vi "站点编码更新（年月日）.vi"(10 "当前编码信息":string, 11 "站别":string) -> ()   [LabVIEW 2018]
uses:
  <vilib>/Utility/file.llb/Read From Spreadsheet File (string).vi
panel:
  out "错误输出":errorcluster
  out "error out":errorcluster caption="错误输出"
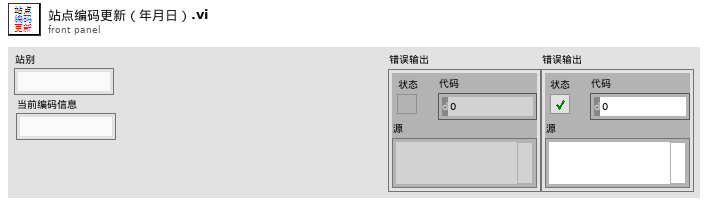
[diagram p1: front panel]
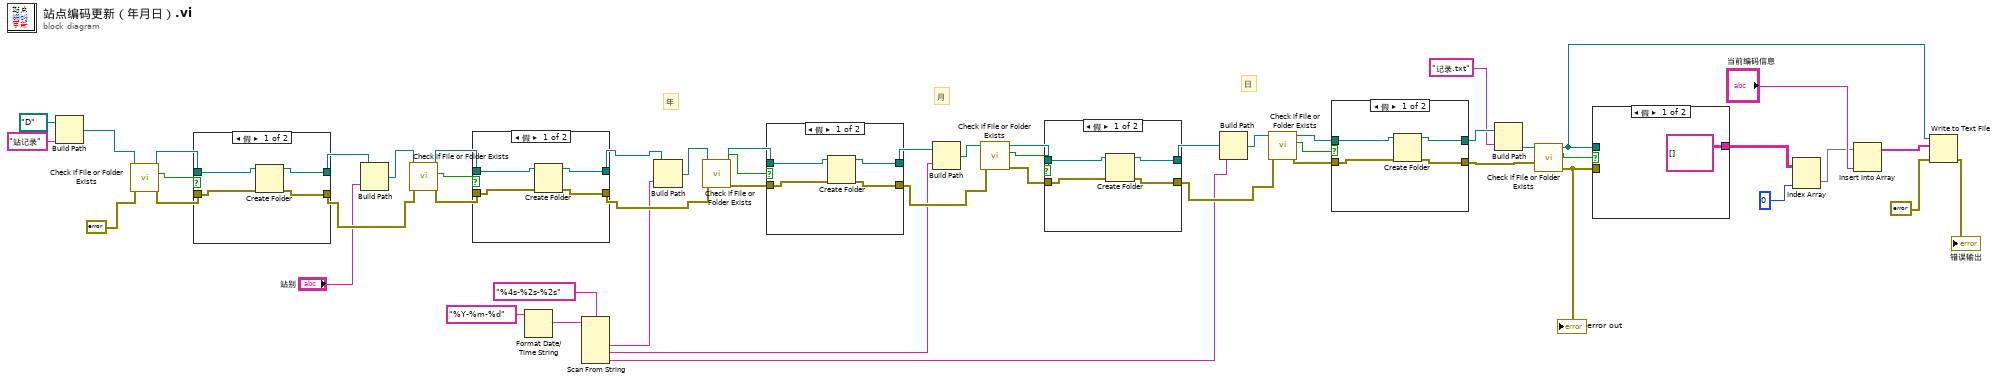
[diagram p0: block diagram]
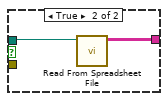
[diagram p2: hidden frame]
diagram:
  # "日"
  # "月"
  # "年"
  n1 = Build Path(base path=path "D:/" ("基路径"), name or relative path="站记录" ("名称或相对路径")) -> (appended path=w50:path)
  n2 = call <vilib>:"Check if File or Folder Exists.vi"("error in (no error)"=errorcluster {"status"=FALSE, "code"=0, "source"=""}, "path"=w50) -> ("error out"=w47:errorcluster, "file or folder exists?"=w49:bool, "dup path"=w48:path)  [unwired: 7 in]
  n3 = case shown="假" w49 {
    tunnel: w48 -> [w56 w58]
    tunnel: w47 -> [w55 w57]
    tunnel: [w54 w58] -> w42
    tunnel: [w53 w57] -> w40
    frame False {
      n4 = Create Folder(path (use dialog)=w56, error in=w55) -> (created path=w54:path, error out=w53:errorcluster)  [unwired: 1 in, 1 out]
    }
    frame True {
    }
  }
  n5 = Build Path(base path=w42, name or relative path="站别") -> (appended path=w41:path)
  n6 = call <vilib>:"Check if File or Folder Exists.vi"("error in (no error)"=w40, "path"=w41) -> ("error out"=w44:errorcluster, "file or folder exists?"=w46:bool, "dup path"=w45:path)  [unwired: 7 in]
  n7 = case shown="假" w46 {
    tunnel: w45 -> [w62 w64]
    tunnel: w44 -> [w61 w63]
    tunnel: [w60 w64] -> w34
    tunnel: [w59 w63] -> w33
    frame False {
      n8 = Create Folder(path (use dialog)=w62, error in=w61) -> (created path=w60:path, error out=w59:errorcluster)  [unwired: 1 in, 1 out]
    }
    frame True {
    }
  }
  n9 = Format Date/Time String(time format string (%c)="%Y-%m-%d" ("时间格式字符串(%c)")) -> (date/time string=w31:string)  [unwired: 2 in]
  n10 = Scan From String(format string="%4s-%2s-%2s" ("格式字符串"), input string=w31) -> (output 1=w29:string, output 2=w22:string, output 3=w15:string)  [unwired: 5 in, 3 out]
  n11 = Build Path(base path=w34, name or relative path=w29) -> (appended path=w35:path)
  n12 = call <vilib>:"Check if File or Folder Exists.vi"("error in (no error)"=w33, "path"=w35) -> ("error out"=w36:errorcluster, "file or folder exists?"=w38:bool, "dup path"=w37:path)  [unwired: 7 in]
  n13 = case shown="假" w38 {
    tunnel: w37 -> [w68 w70]
    tunnel: w36 -> [w67 w69]
    tunnel: [w66 w70] -> w24
    tunnel: [w65 w69] -> w23
    frame False {
      n14 = Create Folder(path (use dialog)=w68, error in=w67) -> (created path=w66:path, error out=w65:errorcluster)  [unwired: 1 in, 1 out]
    }
    frame True {
    }
  }
  n15 = Build Path(base path=w24, name or relative path=w22) -> (appended path=w25:path)
  n16 = call <vilib>:"Check if File or Folder Exists.vi"("error in (no error)"=w23, "path"=w25) -> ("error out"=w26:errorcluster, "file or folder exists?"=w28:bool, "dup path"=w27:path)  [unwired: 7 in]
  n17 = case shown="假" w28 {
    tunnel: w27 -> [w74 w76]
    tunnel: w26 -> [w73 w75]
    tunnel: [w72 w76] -> w16
    tunnel: [w71 w75] -> w17
    frame False {
      n18 = Create Folder(path (use dialog)=w74, error in=w73) -> (created path=w72:path, error out=w71:errorcluster)  [unwired: 1 in, 1 out]
    }
    frame True {
    }
  }
  n19 = Build Path(base path=w16, name or relative path=w15) -> (appended path=w18:path)
  n20 = call <vilib>:"Check if File or Folder Exists.vi"("error in (no error)"=w17, "path"=w18) -> ("error out"=w19:errorcluster, "file or folder exists?"=w21:bool, "dup path"=w20:path)  [unwired: 7 in]
  n21 = case shown="假" w21 {
    tunnel: w20 -> [w80 w82]
    tunnel: w19 -> [w79 w81]
    tunnel: [w78 w82] -> w8
    tunnel: [w77 w81] -> w7
    frame False {
      n22 = Create Folder(path (use dialog)=w80, error in=w79) -> (created path=w78:path, error out=w77:errorcluster)  [unwired: 1 in, 1 out]
    }
    frame True {
    }
  }
  n23 = Build Path(base path=w8, name or relative path="记录.txt" ("名称或相对路径")) -> (appended path=w9:path)
  n24 = call <vilib>:"Check if File or Folder Exists.vi"("error in (no error)"=w7, "path"=w9) -> ("error out"=w10:errorcluster, "file or folder exists?"=w11:bool, "dup path"=w3:path)  [unwired: 7 in]
  "error out" <- w10
  n25 = case shown="假" w11 {
    tunnel: w3 -> [_ w85]
    tunnel: w10 -> [_ _]
    tunnel: [string[][] [] ("all rows") w84] -> w5
    frame False {
    }
    frame True {
      n26 = call-poly <vilib>:"Read From Spreadsheet File.vi"("file path (dialog if empty)"=w85) -> ("all rows"=w84:string[][])  [unwired: 6 in, 4 out]
    }
  }
  n27 = Index Array(array=w5, index (col)=0 ("禁用的索引 (列)")) -> (element=w12:string[])  [unwired: 1 in]
  n28 = Insert Into Array(array=w12, new element="当前编码信息") -> (w4:string[])  [unwired: 1 in]
  n29 = Write to Text File(file (use dialog)=w3, text=w4, error in=errorcluster {"status"=FALSE, "code"=0, "source"=""} ("错误输入")) -> (error out=→"错误输出":errorcluster)  [unwired: 1 in, 2 out]
